vi "CAN BOOT Write App Data.vi"(6 "TimeOutOfMs":u32, 7 "CRC16":u16, 9 "NAD":u8, 10 "CANIndex":i32, 11 "DevHandle":i32) -> (3 "function return":i32)   [LabVIEW 2010, in "can_bootloader.lvlib"]
doc: "int WINAPI CAN_BOOT_WriteAppData(int DevHandle,int CANIndex,unsigned char NAD,unsigned short CRC16,unsigned int TimeOutOfMs);"
uses:
  can_bootloader.lvlib
  USB2XXX/trunk/USB2XXX/USB2XXX/vs2010/Release/USB2XXX.dll
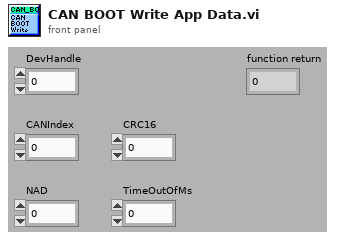
[diagram p1: front panel]
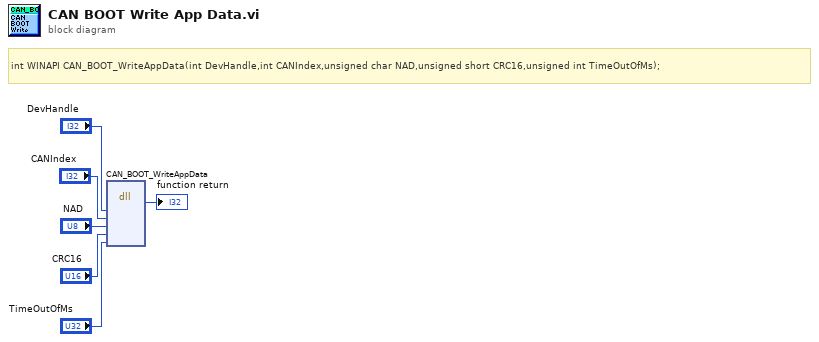
[diagram p0: block diagram]
diagram:
  # "int WINAPI CAN_BOOT_WriteAppData(int DevHandle,int CANIndex,unsigned char NAD,unsigned short CRC16,unsigned int TimeOutOfMs);"
  n1 = dll-call lib="E:/OtherWork/STM32/USB2XXX/trunk/USB2XXX/USB2XXX/vs2010/Release/USB2XXX.*" fn="CAN_BOOT_WriteAppData"("DevHandle"="DevHandle", "CANIndex"="CANIndex", "NAD"="NAD", "CRC16"="CRC16", "TimeOutOfMs"="TimeOutOfMs") -> (→"function return":i32)  [unwired: 8 in, 2 out]
